vi "Example Digital Input Output.vi"() -> ()   [LabVIEW 2015]
panel:
  out "Read value group CH 8 - 15":u64(slide) max=255 step=1 scale=0.0..255.0
  out "Read value group CH 0-7":u64(slide) max=255 step=1 scale=0.0..255.0
  in  "Connect Btn":bool
  in  "Write value group CH 8-15":u64(slide) max=255 step=1 scale=0.0..255.0
  in  "Write value group CH 0-7":u64(slide) max=255 step=1 scale=0.0..255.0
  in  "Calibrate":bool
  in  "Stop Button":bool
  in  "Active ADALM2000 URIs:":u16(ring) items=["ip:192.168.2.1", "usb:2.6.5"]
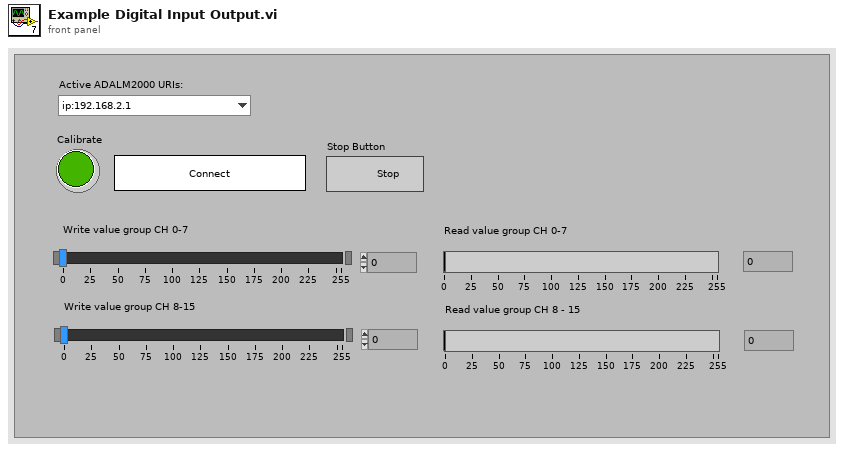
[diagram p1: front panel]
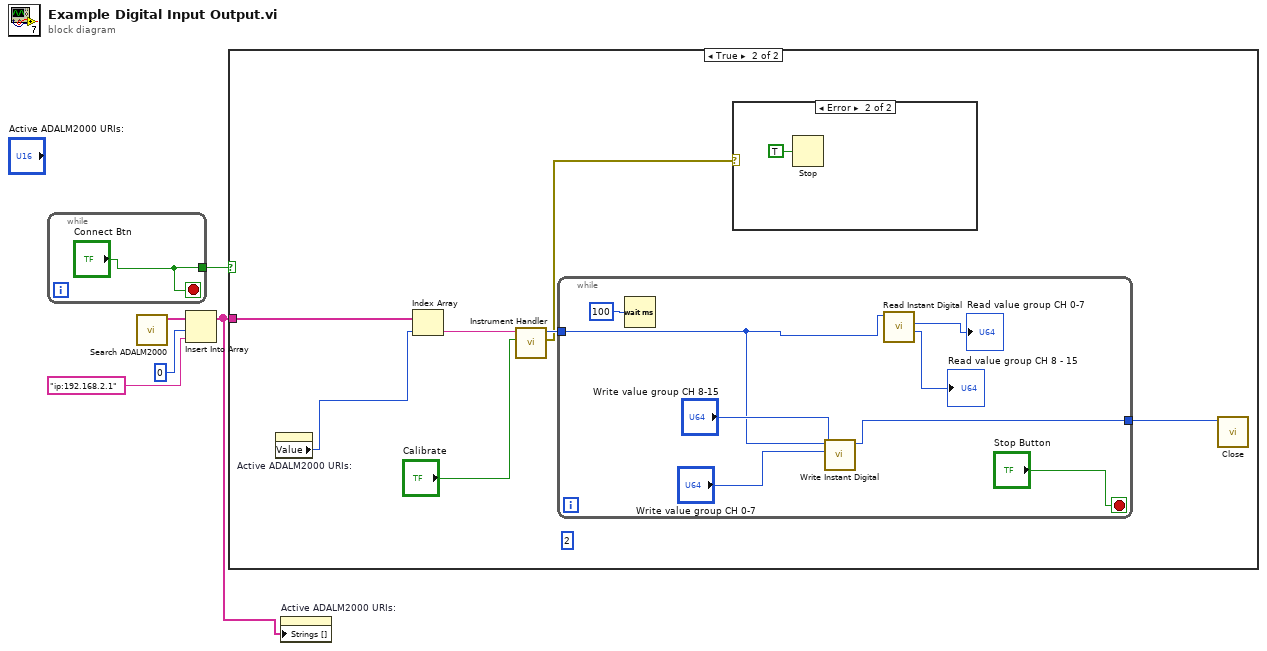
[diagram p0: block diagram]
diagram:
  n1 = while {
    tunnel: ["Connect Btn"] -> w2
    stop <- "Connect Btn" stop-if-true
  }
  n2 = call "Search ADALM2000.vi"() -> ("Array"=w5:string[])  [unwired: 11 in]
  n3 = Insert Into Array(array=w5, index=0, new element="ip:192.168.2.1" ("new element/subarray")) -> (w1:string[])
  n4 = case shown="True" w2 {
    tunnel: w1 -> [_ w13]
    frame False {
    }
    frame True {
      (unwired) 2
      n5 = property on="Active ADALM2000 URIs:" class="Ring (strict)"() -> ("Value"=w9:u16)  [unwired: 2 in, 2 out]
      n6 = Index Array(array=w13, index=w9) -> (element=w12:string)
      n7 = call "Instrument Handler.vi"("Calibrate"="Calibrate", "ADALM2000 URI"=w12) -> ("error out"=w7:errorcluster, "ADALM2000 Handle"=w11:u32)  [unwired: 8 in]
      n8 = while {
        tunnel: w11 -> [w18]
        tunnel: [w17] -> w10
        stop <- "Stop Button" stop-if-true
        n9 = Wait (ms)(milliseconds to wait=u32 100) -> ()  [unwired: 1 out]
        n10 = call "Write Instant Digital.vi"("Write value group CH 8-15"="Write value group CH 8-15", "Write value group CH 0-7"="Write value group CH 0-7", "ADALM2000 Handler"=w18) -> ("ADALM2000 Handler 2"=w17:u32)  [unwired: 8 in]
        n11 = call "Read Instant Digital.vi"("ADALM2000 Handler"=w18) -> ("Read value group CH 8-15"=→"Read value group CH 8 - 15":u64, "Read value group CH 0-7"=→"Read value group CH 0-7":u64)  [unwired: 8 in, 1 out]
      }
      n12 = case shown="Error" w7 {
        frame No Error {
        }
        frame Error {
          n13 = Stop(stop? (T)=TRUE) -> ()
        }
      }
      n14 = call "Close.vi"("ADALM2000 Handler"=w10) -> ()  [unwired: 11 in]
    }
  }
  n15 = property on="Active ADALM2000 URIs:" class="Ring (strict)"("Strings []"=w1) -> ()  [unwired: 2 in, 2 out]
